vi "[RT] Cont Acq wPause.vi"() -> ()   [LabVIEW 2015]
doc: "If a finite acquisition is too large for the amount of memory available on the host controller, then perform a continuous acquisition for a finite period of time. When you call rwfm_Stop.vi, the FPGA stops the acquisition and immediately rearms itself waiting for rwfm_Start.vi to be called. The stop VI also flushes the host application's data buffer so subsequent acquisitions do not return old data."
uses:
  <vilib>/rvi/interface/nirviCloseFPGA/nirviCloseFPGA.xnode
  <vilib>/NI/cRIO Wfm/cRIO Wfm.lvlib
  <vilib>/NI/cRIO Wfm/AcqRead(Wfm).vi
  <vilib>/rvi/interface/nirviOpenFPGA/nirviOpenFPGA.xnode
  <vilib>/FPGAPlugInAG/cRIO-9074/niLvFpga_Open_cRIO-9074.vi
  <vilib>/rvi/interface/common/dynamic/niFpgaDynamicAddResources.vi
  <vilib>/FPGAPlugInAG/Dynamic/niLvFpga_Close_Dynamic.vi
  C:/Program Files (x86)/National Instruments/LabVIEW 2015/ProjectTemplates/Source/cRIOWfm/FPGA Bitfiles/DeltaSigMain_9074.lvbitx
  C:/Program Files (x86)/National Instruments/LabVIEW 2015/ProjectTemplates/Source/cRIOWfm/FPGA/[FPGA] DeltaSig Main.vi
  C:/Program Files (x86)/National Instruments/LabVIEW 2015/ProjectTemplates/Source/cRIOWfm/FPGA Bitfiles/SARAcqMain_9074.lvbitx
  C:/Program Files (x86)/National Instruments/LabVIEW 2015/ProjectTemplates/Source/cRIOWfm/FPGA/[FPGA] SAR Acq Main.vi
  <vilib>/NI/cRIO Wfm/ChannelConfig.ctl
panel:
  in  "Sample Rate":u32=51200
  in  "Channel Info":T1=[{"Channel Name"="Mod1/ai0", "Sensitivity mV_EU"=1000.0, "EU"="V", "dB Ref EU"=1.0}, {"Channel Name"="Mod1/ai1", "Sensitivity mV_EU"=1000.0, "EU"="V", "dB Ref EU"=1.0}, {"Channel Name"="Mod1/ai2", "Sensitivity mV_EU"=1000.0, "EU"="V", "dB Ref EU"=1.0}, {"Channel Name"="Mod1/ai3", "Sensitivity mV_EU"=1000.0, "EU"="V", "dB Ref EU"=1.0}] caption="Channel Name      Scale [mV/EU]        EU           dB Ref [EU]" {"dB Ref EU" format="%#.2p"; "Sensitivity mV_EU" format="%.2f"}
  in  "Samps per Chan":i32=25600 caption="Samples per Channel"
  out "RT Buffer Backlog [%]":dbl format="%#.2g"
  in  "Pause":bool
  out "Waveform Graph":waveform(sgl)[](graph)
  in  "stop":bool
  # "Sampling Info"
  # "Channel Info"
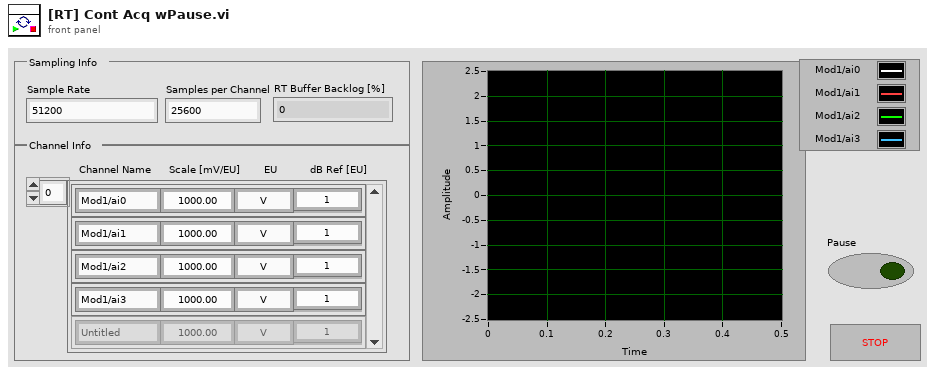
[diagram p1: front panel]
types:
  T1 = typedef "cRIO Wfm.lvlib/ChannelConfig.ctl" = cluster{"Channel Name":string, "Sensitivity mV_EU":dbl, "EU":string, "dB Ref EU":dbl}[]
  T2 = typedef "cRIO Wfm.lvlib/SamplingInfo.ctl" = cluster{"Number of Channels":i32, "Actual Samp Rate":dbl, "Chan Name Array":string[], "EU Chan Array":string[], "dB Ref Chan Array":dbl[]}
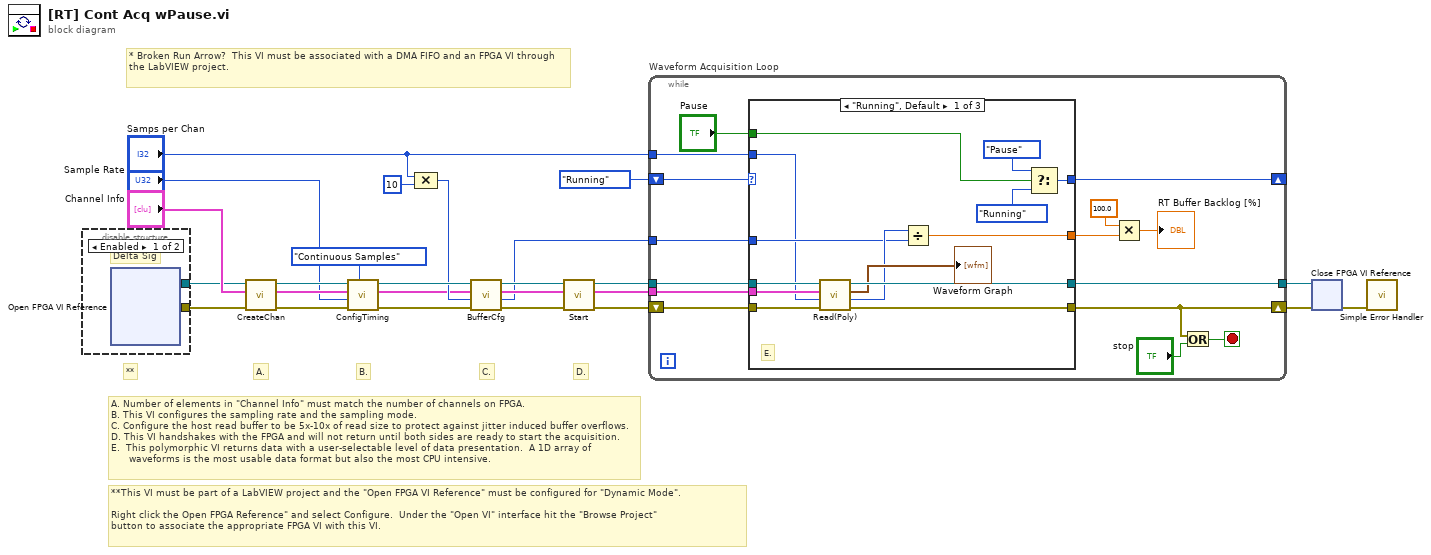
[diagram p0: block diagram]
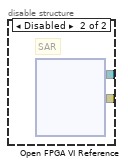
[diagram p2: hidden frame]
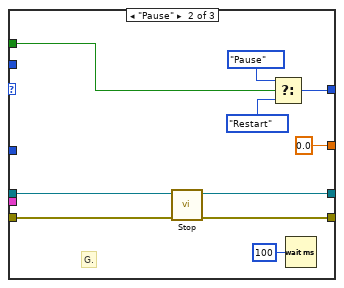
[diagram p3: hidden frame]
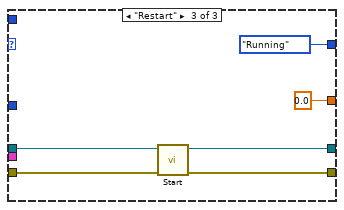
[diagram p4: hidden frame]
diagram:
  # "**This VI must be part of a LabVIEW project and the \"Open FPGA VI Reference\" must be configured for \"Dynamic Mode\".\n\nRight click the Open FPGA Reference\" and select Configure.  Under the \"Open VI\" interface hit the \"Browse Project\" \nbutton to associate the appropriate FPGA VI with this VI."
  # "* Broken Run Arrow?  This VI must be associated with a DMA FIFO and an FPGA VI through the LabVIEW project."
  # "**"
  # "D."
  # "C."
  # "B."
  # "A."
  # "A. Number of elements in \"Channel Info\" must match the number of channels on FPGA.\nB. This VI configures the sampling rate and the sampling mode.\nC. Configure the host read buffer to be 5x-10x of read size to protect against jitter induced buffer overflows.\nD. This VI handshakes with the FPGA and will not return until both sides are ready to start the acquisition.\nE.  This polymorphic VI returns data with a user-selectable level of data presentation.  A 1D array of     \n      waveforms is the most usable data format but also the most CPU intensive."
  n1 = disable-structure shown="Enabled" {
    disable-tunnel: [w27 w29] -> w2
    disable-tunnel: [w26 w28] -> w1
    frame Enabled {
      # "Delta Sig"
      n2 = xnode "Open FPGA VI Reference"() -> ("FPGA VI Reference Out"=w27:refnum<k20>, "error out"=w26:errorcluster)  [unwired: 2 in]
    }
    frame Disabled {
      # "SAR"
      n3 = xnode "Open FPGA VI Reference"() -> ("FPGA VI Reference Out"=w29:refnum<k20>, "error out"=w28:errorcluster)  [unwired: 2 in]
    }
  }
  n4 = call <vilib>:"CreateChan.vi"("error in"=w1, "Channel Info"="Channel Info", "Dynamic FPGA Ref"=w2) -> ("error out"=w11:errorcluster, "Sampling Info"=w10:T2, "Dynamic FPGA Ref Out"=w12:refnum<k20>)  [unwired: 1 in, 5 out]
  n5 = call <vilib>:"ConfigTiming.vi"("Sample Mode"=enum16{"Finite Samples", "Continuous Samples"}."Continuous Samples", "error in"=w11, "Sample Rate"="Sample Rate", "Sampling Info In"=w10, "Dynamic FPGA Ref"=w12) -> ("error out"=w20:errorcluster, "Sampling Info Out"=w9:T2, "Dynamic FPGA Ref Out"=w21:refnum<k20>)  [unwired: 3 in, 1 out]
  n6 = Compound Arithmetic op=MULTIPLY("Samps per Chan", 10 ("value")) -> (w13:i32)
  n7 = call <vilib>:"BufferCfg.vi"("error in"=w20, "Buffer Size [Samps per Chan]"=w13, "Sampling Info In"=w9, "Dynamic FPGA Ref"=w21) -> ("error out"=w15:errorcluster, "Buffer Size [Total Samples]"=w6:u32, "Sampling Info Out"=w8:T2, "Dynamic FPGA Ref Out"=w16:refnum<k20>)  [unwired: 4 out]
  n8 = call <vilib>:"Start.vi"("error in"=w15, "Sampling Info In"=w8, "Dynamic FPGA Ref"=w16) -> ("error out"=w24:errorcluster, "Sampling Info Out"=w7:T2, "Dynamic FPGA Ref Out"=w25:refnum<k20>)  [unwired: 6 out]
  n9 = while "Waveform Acquisition Loop" {
    tunnel: w25 -> [w43]
    tunnel: [w40] -> w23
    shift-right: [w38] -> _
    shift-left: enum16{"Running", "Pause", "Restart"}."Running" ("ReadCmnd") -> [w39]
    tunnel: w7 -> [w36]
    tunnel: w6 -> [w35]
    tunnel: "Samps per Chan" -> [w31]
    shift-right: [w30] -> w22
    shift-left: w24 -> [w41]
    stop <- w42 stop-if-true
    n10 = case shown="\"Running\", Default" w39 {
      tunnel: w43 -> [w58 w64 w74]
      tunnel: w41 -> [w57 w63 w73]
      tunnel: [w56 w62 w72] -> w40
      tunnel: [w55 w61 w71] -> w30
      tunnel: [w54 w66 enum16{"Running", "Pause", "Restart"}."Running" ("ReadCmnd")] -> w38
      tunnel: "Pause" -> [w51 w65 _]
      tunnel: w36 -> [w50 _ _]
      tunnel: w35 -> [w47 _ _]
      tunnel: [w46 0.0 0.0] -> w32
      tunnel: w31 -> [w45 _ _]
      frame "Running", Default {
        # "E."
        n11 = call-poly <vilib>:"Read(Poly).vi"("error in"=w57, "Samps Read per Chan"=w45, "Sampling Info"=w50, "Dynamic FPGA Ref"=w58) -> ("error out"=w55:errorcluster, "Samples Remaining"=w48:u32, "Wfm Data"=→"Waveform Graph":waveform(sgl)[], "Dynamic FPGA Ref Out"=w56:refnum<k20>)  [unwired: 2 in, 2 out]
        n12 = Divide(x=w48, y=w47) -> (x/y=w46:dbl)
        n13 = Select(t=enum16{"Running", "Pause", "Restart"}."Pause" ("ReadCmnd"), s=w51, f=enum16{"Running", "Pause", "Restart"}."Running" ("ReadCmnd")) -> (s? t:f=w54:enum16{"Running", "Pause", "Restart"})
      }
      frame "Pause" {
        # "G."
        n14 = call <vilib>:"Stop.vi"("error in"=w63, "Dynamic FPGA Ref"=w64) -> ("error out"=w61:errorcluster, "Dynamic FPGA Ref Out"=w62:refnum<k20>)  [unwired: 8 out]
        n15 = Select(t=enum16{"Running", "Pause", "Restart"}."Pause" ("ReadCmnd"), s=w65, f=enum16{"Running", "Pause", "Restart"}."Restart" ("ReadCmnd")) -> (s? t:f=w66:enum16{"Running", "Pause", "Restart"})
        n16 = Wait (ms)(milliseconds to wait=u32 100) -> ()  [unwired: 1 out]
      }
      frame "Restart" {
        n17 = call <vilib>:"Start.vi"("error in"=w73, "Dynamic FPGA Ref"=w74) -> ("error out"=w71:errorcluster, "Dynamic FPGA Ref Out"=w72:refnum<k20>)  [unwired: 1 in, 7 out]
      }
    }
    n18 = Multiply(x=100.0, y=w32) -> (x*y=→"RT Buffer Backlog [%]":dbl)
    n19 = Or(x=w30, y="stop") -> (x .or. y?=w42:bool)
  }
  n20 = xnode "Close FPGA VI Reference"("FPGA VI Reference In"=w23, "error in"=w22) -> ("error out"=w18:errorcluster)
  n21 = call <vilib>:"Simple Error Handler.vi"("error in (no error)"=w18) -> ()  [unwired: 1 in, 8 out]
